vi "video.update_free.vi"(8 "error in":errorcluster, 11 "VideoUpdateStaging in":refnum<class "VideoUpdateStaging.lvclass">) -> (0 "error out":errorcluster, 3 "VideoUpdateStaging out":refnum<class "VideoUpdateStaging.lvclass">)   [LabVIEW 2020, in "VideoUpdateStaging.lvclass"]
doc: "Releases the handle and its associated resources."
uses:
  VideoUpdateStaging.lvclass
  VideoUpdateStaging.lvclass/VideoUpdateStaging.ctl
  client.lvlib
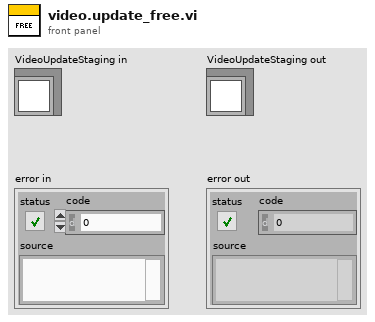
[diagram p1: front panel]
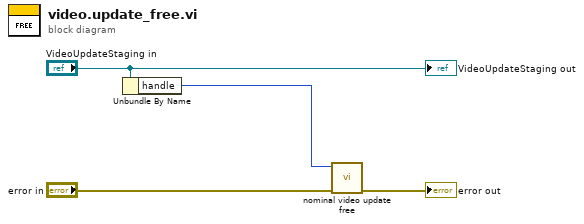
[diagram p0: block diagram]
diagram:
  n1 = Unbundle By Name("VideoUpdateStaging in") -> ("handle"=w2:i32)
  n2 = call "nominal video update free.vi"("error in (no error)"="error in", "staging"=w2) -> ("error out"=→"error out":errorcluster)  [unwired: 8 in, 1 out]
  "VideoUpdateStaging out" <- "VideoUpdateStaging in"
